vi "Validate.vi"(8 "error in":errorcluster, 10 "parameters":variant, 11 "Repository in":refnum<class "NISE_CEF_Repository.lvclass">) -> (0 "error out":errorcluster, 3 "Repository out":refnum<class "NISE_CEF_Repository.lvclass">)   [LabVIEW 2013, in "NISE_CEF_Repository.lvclass"]
doc: "An abstract method for validating the information inside of a repo is accurate. This method should be called before saving the information to file."
uses:
  NISE_CEF_Repository.lvclass
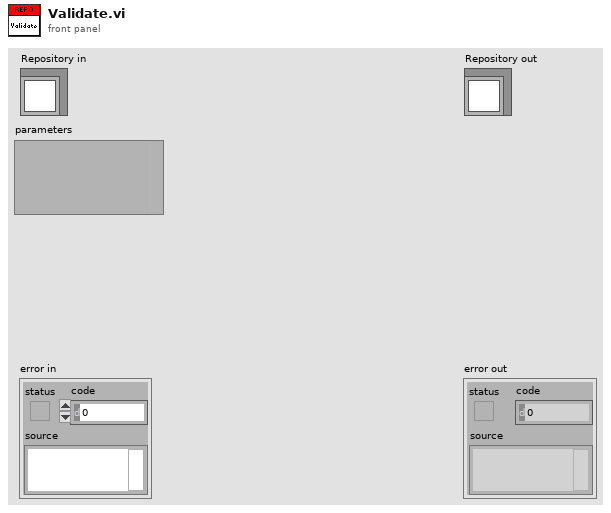
[diagram p1: front panel]
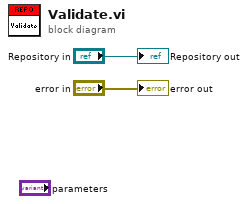
[diagram p0: block diagram]
diagram:
  "error out" <- "error in"
  "Repository out" <- "Repository in"
